vi "VArray to column named VCluster.vi"(8 "error in (no error)":errorcluster, 10 "columns":string[](array[string]), 11 "data":variant) -> (0 "error out":errorcluster, 3 "data (Cluster)":variant)   [LabVIEW 2020, in "Database Reuse.lvlib"]
uses:
  Database Reuse.lvlib
  <vilib>/Utility/Data Type/NI_Data Type.lvlib
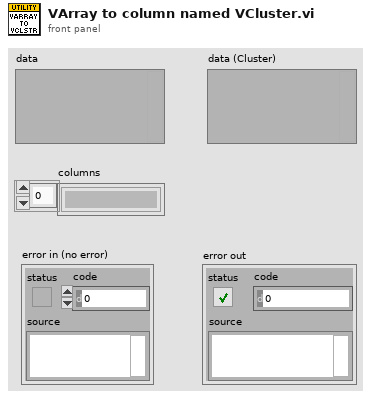
[diagram p1: front panel]
types:
  T1 = typedef "NI_Data Type.lvlib/Data Type.ctl" = enum8{"Invalid Type", "Void", "I8", "I16", "I32", "I64", "U8", "U16", "U32", "U64", "Single Float", "Double Float", "Extended Float", "Single Complex", "Double Complex", "Extended Complex", "Enum U8", "Enum U16", "Enum U32", "Enum U64", "Single Float With Unit", "Double Float With Unit", "Extended Float With Unit", "Single Complex with Unit", "Double Complex with Unit", "Extended Complex with Unit", "Boolean", "String", "Path", "Picture", "Tag", "Array", "Cluster", "Variant", "LV Variant", "Waveform", "Timestamp", "Digital Waveform", "Digital Data", "ExpressData", "Refnum", "External Data", "VI", "Poly VI", "LabVIEW Class Instance", "Fixed Point", "Set Collection", "Map Collection"}
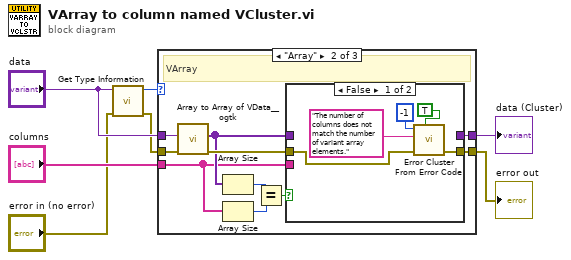
[diagram p0: block diagram]
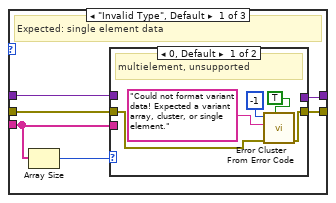
[diagram p2: hidden frame]
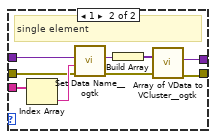
[diagram p3: hidden frame]
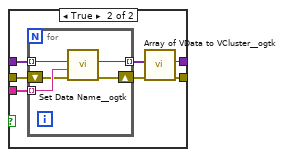
[diagram p4: hidden frame]
diagram:
  n1 = call <vilib>:"Get Type Information.vi"("error in (no error)"="error in (no error)", "variant"="data") -> ("error out"=w3:errorcluster, "type"=w7:T1)  [unwired: 5 in, 3 out]
  n2 = case shown="\"Array\"" w7 {
    tunnel: "data" -> [w12 w37 w56]
    tunnel: [w8 w36 w56] -> w4
    tunnel: "columns" -> [w11 w31 _]
    tunnel: w3 -> [w10 w35 w55]
    tunnel: [w9 w33 w55] -> w1
    frame "Invalid Type", Default {
      # "Expected: single element data"
      n3 = Array Size(array=w11) -> (size(s)=w13:i32)
      n4 = case shown="0, Default" w13 {
        tunnel: w12 -> [_ w25]
        tunnel: w11 -> [_ w27]
        tunnel: w10 -> [w15 w24]
        tunnel: [w14 w20] -> w9
        tunnel: [_ w21] -> w8
        frame 0, Default {
          # "multielement, unsupported"
          n5 = call <vilib>:"Error Cluster From Error Code.vi"("show call chain? (False)"=TRUE, "error in (no error)"=w15, "error message (\"\")"="Could not format variant data! Expected a variant array, cluster, or single element.", "error code (0)"=-1) -> ("error out"=w14:errorcluster)  [unwired: 5 in]
        }
        frame 1 {
          # "single element"
          n6 = Index Array(array=w27) -> (element=w26:string)  [unwired: 1 in]
          n7 = call <userlib>:"Set Data Name__ogtk.vi"("error in (no error)"=w24, "Data Name"=w26, "Data"=w25) -> ("error out"=w19:errorcluster, "Renamed Data"=w23:variant)  [unwired: 7 in]
          n8 = Build Array(w23) -> (w22:variant[])
          n9 = call <userlib>:"Array of VData to VCluster__ogtk.vi"("error in (no error)"=w19, "Array"=w22) -> ("error out"=w20:errorcluster, "VCluster"=w21:variant)  [unwired: 8 in]
        }
      }
    }
    frame "Array" {
      # "VArray"
      n10 = call <userlib>:"Array to Array of VData__ogtk.vi"("error in (no error)"=w35, "MultiD Array"=w37) -> ("error out"=w34:errorcluster, "1D Array of Variants"=w32:variant[])  [unwired: 8 in]
      n11 = Array Size(array=w32) -> (size(s)=w29:i32)
      n12 = Array Size(array=w31) -> (size(s)=w30:i32)
      n13 = Equal?(x=w29, y=w30) -> (x = y?=w28:bool)
      n14 = case shown="False" w28 {
        tunnel: [_ w48] -> w36
        tunnel: w34 -> [w39 w47]
        tunnel: [w40 w45] -> w33
        tunnel: w32 -> [_ w44]
        tunnel: w31 -> [_ w43]
        frame False {
          n15 = call <vilib>:"Error Cluster From Error Code.vi"("show call chain? (False)"=TRUE, "error in (no error)"=w39, "error message (\"\")"="The number of columns does not match the number of variant array elements.", "error code (0)"=-1) -> ("error out"=w40:errorcluster)  [unwired: 5 in]
        }
        frame True {
          n16 = for {
            tunnel: w44 -> [w54] mode=indexing
            tunnel: w43 -> [w53] mode=indexing
            tunnel: [w52] -> w49 mode=indexing
            shift-right: [w50] -> w46
            shift-left: w47 -> [w51]
            n17 = call <userlib>:"Set Data Name__ogtk.vi"("error in (no error)"=w51, "Data Name"=w53, "Data"=w54) -> ("error out"=w50:errorcluster, "Renamed Data"=w52:variant)  [unwired: 7 in]
          }
          n18 = call <userlib>:"Array of VData to VCluster__ogtk.vi"("error in (no error)"=w46, "Array"=w49) -> ("error out"=w45:errorcluster, "VCluster"=w48:variant)  [unwired: 8 in]
        }
      }
    }
    frame "Cluster" {
      # "Already a cluster--no change"
    }
  }
  "data (Cluster)" <- w4
  "error out" <- w1
